vi "VI Tree.vi"   [LabVIEW 2012, in "Tektronix TTR500 Series.lvlib"]
doc: "This is the instrument driver for the Tektronix TTR500 Series RF Network Analyzer. The VI Tree displays all the user-callable VIs of the instrument driver in an organized table."
uses:
  <instrlib>/Tektronix TTR500 Series/Tektronix TTR500 Series.lvlib
panel:
  # "Tektronix TTR500 Series Tree"
  # "SEE DIAGRAM\nFOR VI TREE."
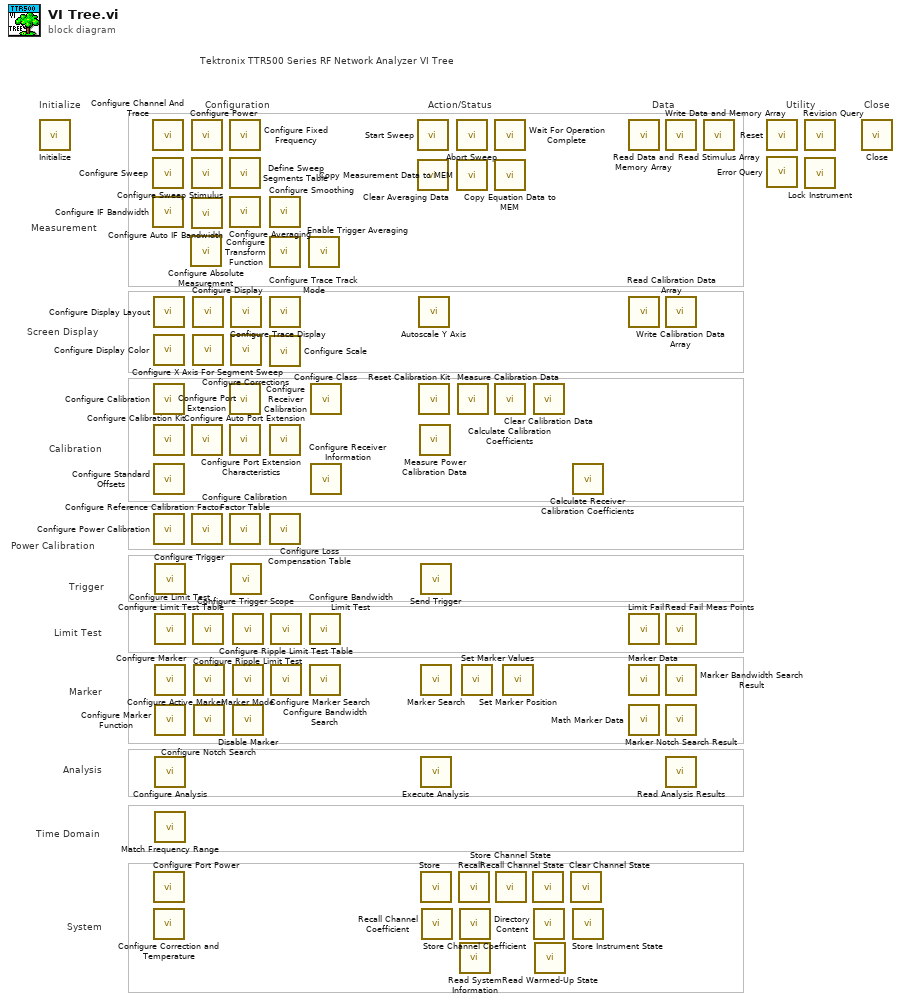
[diagram p0: block diagram]
diagram:
  # "Time Domain"
  # "System"
  # "Analysis"
  # "Marker"
  # "Limit Test"
  # "Trigger"
  # "Power Calibration"
  # "Tektronix TTR500 Series RF Network Analyzer VI Tree"
  # "Calibration"
  # "Screen Display"
  # "Measurement"
  # "Configuration"
  # "Utility"
  # "Data"
  # "Action/Status"
  # "Close"
  # "Initialize"
  n1 = call <instrlib>:"Initialize.vi"() -> ()  [unwired: 9 in, 3 out]
  n2 = call <instrlib>:"Configure Channel And Trace.vi"() -> ()  [unwired: 10 in, 2 out]
  n3 = call <instrlib>:"Configure Sweep.vi"() -> ()  [unwired: 14 in, 2 out]
  n4 = call <instrlib>:"Configure IF Bandwidth.vi"() -> ()  [unwired: 10 in, 2 out]
  n5 = call <instrlib>:"Configure Display Layout.vi"() -> ()  [unwired: 10 in, 2 out]
  n6 = call <instrlib>:"Configure Display Color.vi"() -> ()  [unwired: 14 in, 2 out]
  n7 = call <instrlib>:"Configure Calibration.vi"() -> ()  [unwired: 18 in, 2 out]
  n8 = call <instrlib>:"Configure Calibration Kit.vi"() -> ()  [unwired: 26 in, 2 out]
  n9 = call <instrlib>:"Configure Standard Offsets.vi"() -> ()  [unwired: 10 in, 2 out]
  n10 = call <instrlib>:"Configure Power Calibration.vi"() -> ()  [unwired: 14 in, 2 out]
  n11 = call <instrlib>:"Configure Port Power.vi"() -> ()  [unwired: 10 in, 2 out]
  n12 = call <instrlib>:"Configure Correction and Temperature.vi"() -> ()  [unwired: 10 in, 2 out]
  n13 = call <instrlib>:"Configure Trigger.vi"() -> ()  [unwired: 10 in, 2 out]
  n14 = call <instrlib>:"Configure Limit Test.vi"() -> ()  [unwired: 10 in, 2 out]
  n15 = call <instrlib>:"Configure Marker.vi"() -> ()  [unwired: 10 in, 2 out]
  n16 = call <instrlib>:"Configure Marker Function.vi"() -> ()  [unwired: 10 in, 2 out]
  n17 = call <instrlib>:"Configure Analysis.vi"() -> ()  [unwired: 18 in, 2 out]
  n18 = call <instrlib>:"Match Frequency Range.vi"() -> ()  [unwired: 14 in, 2 out]
  n19 = call <instrlib>:"Configure Absolute Measurement.vi"() -> ()  [unwired: 14 in, 2 out]
  n20 = call <instrlib>:"Configure Power.vi"() -> ()  [unwired: 14 in, 2 out]
  n21 = call <instrlib>:"Configure Sweep Stimulus.vi"() -> ()  [unwired: 10 in, 2 out]
  n22 = call <instrlib>:"Configure Auto IF Bandwidth.vi"() -> ()  [unwired: 10 in, 2 out]
  n23 = call <instrlib>:"Configure Port Extension.vi"() -> ()  [unwired: 10 in, 2 out]
  n24 = call <instrlib>:"Configure Reference Calibration Factor.vi"() -> ()  [unwired: 14 in, 2 out]
  n25 = call <instrlib>:"Configure Display.vi"() -> ()  [unwired: 26 in, 2 out]
  n26 = call <instrlib>:"Configure X Axis For Segment Sweep.vi"() -> ()  [unwired: 10 in, 2 out]
  n27 = call <instrlib>:"Configure Limit Test Table.vi"() -> ()  [unwired: 14 in, 2 out]
  n28 = call <instrlib>:"Configure Active Marker.vi"() -> ()  [unwired: 10 in, 2 out]
  n29 = call <instrlib>:"Configure Notch Search.vi"() -> ()  [unwired: 10 in, 2 out]
  n30 = call <instrlib>:"Configure Fixed Frequency.vi"() -> ()  [unwired: 10 in, 2 out]
  n31 = call <instrlib>:"Define Sweep Segments Table.vi"() -> ()  [unwired: 18 in, 2 out]
  n32 = call <instrlib>:"Configure Averaging.vi"() -> ()  [unwired: 10 in, 2 out]
  n33 = call <instrlib>:"Configure Receiver Calibration.vi"() -> ()  [unwired: 10 in, 2 out]
  n34 = call <instrlib>:"Configure Auto Port Extension.vi"() -> ()  [unwired: 10 in, 2 out]
  n35 = call <instrlib>:"Configure Calibration Factor Table.vi"() -> ()  [unwired: 10 in, 2 out]
  n36 = call <instrlib>:"Configure Trace Display.vi"() -> ()  [unwired: 14 in, 2 out]
  n37 = call <instrlib>:"Configure Corrections.vi"() -> ()  [unwired: 14 in, 2 out]
  n38 = call <instrlib>:"Configure Trigger Scope.vi"() -> ()  [unwired: 10 in, 2 out]
  n39 = call <instrlib>:"Configure Ripple Limit Test.vi"() -> ()  [unwired: 10 in, 2 out]
  n40 = call <instrlib>:"Marker Mode.vi"() -> ()  [unwired: 10 in, 2 out]
  n41 = call <instrlib>:"Disable Marker.vi"() -> ()  [unwired: 10 in, 2 out]
  n42 = call <instrlib>:"Configure Smoothing.vi"() -> ()  [unwired: 10 in, 2 out]
  n43 = call <instrlib>:"Configure Transform Function.vi"() -> ()  [unwired: 10 in, 2 out]
  n44 = call <instrlib>:"Configure Trace Track Mode.vi"() -> ()  [unwired: 10 in, 2 out]
  n45 = call <instrlib>:"Configure Scale.vi"() -> ()  [unwired: 14 in, 2 out]
  n46 = call <instrlib>:"Configure Port Extension Characteristics.vi"() -> ()  [unwired: 14 in, 2 out]
  n47 = call <instrlib>:"Configure Loss Compensation Table.vi"() -> ()  [unwired: 10 in, 2 out]
  n48 = call <instrlib>:"Configure Ripple Limit Test Table.vi"() -> ()  [unwired: 14 in, 2 out]
  n49 = call <instrlib>:"Configure Marker Search.vi"() -> ()  [unwired: 18 in, 2 out]
  n50 = call <instrlib>:"Enable Trigger Averaging.vi"() -> ()  [unwired: 10 in, 2 out]
  n51 = call <instrlib>:"Configure Bandwidth Limit Test.vi"() -> ()  [unwired: 14 in, 2 out]
  n52 = call <instrlib>:"Configure Bandwidth Search.vi"() -> ()  [unwired: 10 in, 2 out]
  n53 = call <instrlib>:"Configure Class.vi"() -> ()  [unwired: 10 in, 2 out]
  n54 = call <instrlib>:"Configure Receiver Information.vi"() -> ()  [unwired: 10 in, 2 out]
  n55 = call <instrlib>:"Start Sweep.vi"() -> ()  [unwired: 10 in, 2 out]
  n56 = call <instrlib>:"Clear Averaging Data.vi"() -> ()  [unwired: 10 in, 2 out]
  n57 = call <instrlib>:"Autoscale Y Axis.vi"() -> ()  [unwired: 10 in, 2 out]
  n58 = call <instrlib>:"Reset Calibration Kit.vi"() -> ()  [unwired: 10 in, 2 out]
  n59 = call <instrlib>:"Measure Power Calibration Data.vi"() -> ()  [unwired: 10 in, 2 out]
  n60 = call <instrlib>:"Send Trigger.vi"() -> ()  [unwired: 10 in, 2 out]
  n61 = call <instrlib>:"Marker Search.vi"() -> ()  [unwired: 7 in, 5 out]
  n62 = call <instrlib>:"Execute Analysis.vi"() -> ()  [unwired: 10 in, 2 out]
  n63 = call <instrlib>:"Store.vi"() -> ()  [unwired: 10 in, 2 out]
  n64 = call <instrlib>:"Recall Channel Coefficient.vi"() -> ()  [unwired: 10 in, 2 out]
  n65 = call <instrlib>:"Abort Sweep.vi"() -> ()  [unwired: 10 in, 2 out]
  n66 = call <instrlib>:"Copy Measurement Data to MEM.vi"() -> ()  [unwired: 10 in, 2 out]
  n67 = call <instrlib>:"Measure Calibration Data.vi"() -> ()  [unwired: 10 in, 2 out]
  n68 = call <instrlib>:"Recall.vi"() -> ()  [unwired: 10 in, 2 out]
  n69 = call <instrlib>:"Store Channel Coefficient.vi"() -> ()  [unwired: 10 in, 2 out]
  n70 = call <instrlib>:"Read System Information.vi"() -> ()  [unwired: 6 in, 6 out]
  n71 = call <instrlib>:"Set Marker Values.vi"() -> ()  [unwired: 10 in, 2 out]
  n72 = call <instrlib>:"Wait For Operation Complete.vi"() -> ()  [unwired: 10 in, 2 out]
  n73 = call <instrlib>:"Copy Equation Data to MEM.vi"() -> ()  [unwired: 10 in, 2 out]
  n74 = call <instrlib>:"Calculate Calibration Coefficients.vi"() -> ()  [unwired: 10 in, 2 out]
  n75 = call <instrlib>:"Store Channel State.vi"() -> ()  [unwired: 10 in, 2 out]
  n76 = call <instrlib>:"Set Marker Position.vi"() -> ()  [unwired: 10 in, 2 out]
  n77 = call <instrlib>:"Recall Channel State.vi"() -> ()  [unwired: 10 in, 2 out]
  n78 = call <instrlib>:"Clear Calibration Data.vi"() -> ()  [unwired: 10 in, 2 out]
  n79 = call <instrlib>:"Directory Content.vi"() -> ()  [unwired: 6 in, 6 out]
  n80 = call <instrlib>:"Read Warmed-Up State.vi"() -> ()  [unwired: 9 in, 3 out]
  n81 = call <instrlib>:"Clear Channel State.vi"() -> ()  [unwired: 10 in, 2 out]
  n82 = call <instrlib>:"Calculate Receiver Calibration Coefficients.vi"() -> ()  [unwired: 10 in, 2 out]
  n83 = call <instrlib>:"Store Instrument State.vi"() -> ()  [unwired: 10 in, 2 out]
  n84 = call <instrlib>:"Read Data and Memory Array.vi"() -> ()  [unwired: 8 in, 4 out]
  n85 = call <instrlib>:"Read Calibration Data Array.vi"() -> ()  [unwired: 9 in, 3 out]
  n86 = call <instrlib>:"Limit Fail.vi"() -> ()  [unwired: 9 in, 3 out]
  n87 = call <instrlib>:"Marker Data.vi"() -> ()  [unwired: 7 in, 5 out]
  n88 = call <instrlib>:"Math Marker Data.vi"() -> ()  [unwired: 6 in, 6 out]
  n89 = call <instrlib>:"Write Data and Memory Array.vi"() -> ()  [unwired: 10 in, 2 out]
  n90 = call <instrlib>:"Write Calibration Data Array.vi"() -> ()  [unwired: 10 in, 2 out]
  n91 = call <instrlib>:"Read Fail Meas Points.vi"() -> ()  [unwired: 8 in, 4 out]
  n92 = call <instrlib>:"Marker Bandwidth Search Result.vi"() -> ()  [unwired: 6 in, 6 out]
  n93 = call <instrlib>:"Marker Notch Search Result.vi"() -> ()  [unwired: 6 in, 6 out]
  n94 = call <instrlib>:"Read Analysis Results.vi"() -> ()  [unwired: 7 in, 5 out]
  n95 = call <instrlib>:"Read Stimulus Array.vi"() -> ()  [unwired: 9 in, 3 out]
  n96 = call <instrlib>:"Reset.vi"() -> ()  [unwired: 10 in, 2 out]
  n97 = call <instrlib>:"Error Query.vi"() -> ()  [unwired: 8 in, 4 out]
  n98 = call <instrlib>:"Revision Query.vi"() -> ()  [unwired: 8 in, 4 out]
  n99 = call <instrlib>:"Lock Instrument.vi"() -> ()  [unwired: 10 in, 2 out]
  n100 = call <instrlib>:"Close.vi"() -> ()  [unwired: 11 in, 1 out]
